vi "Initialize and Enable.vi"(4 "error in (no error)":errorcluster, 7 "axis names":string[](array[string])=["Y", "YY", "X", "Z", "U"]) -> (0 "error out":errorcluster, 3 "controller out":refnum<k24>)   [LabVIEW 2011]
uses:
  C:/Users/Admin/Desktop/Gantry Code Transfer/source/Code Transfer/Aerotech.A3200.dll
  Aerotech.A3200.dll
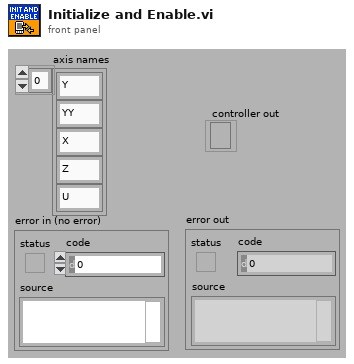
[diagram p1: front panel]
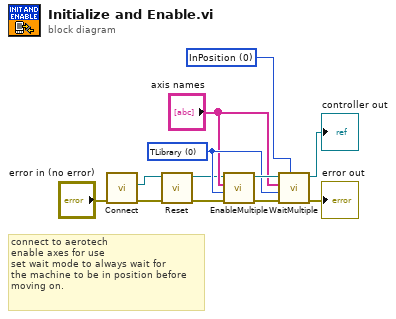
[diagram p0: block diagram]
diagram:
  w11 = 0 items=["InPosition", "MoveDone"] ("wait option?")
  w6 = 0 items=["TLibrary", "T01", "T02", "T03", "T04", "T05", "T06", "T07", "T08", "T09", "T10", "T11", "T12", "T13", "T14", "T15", "T16", "T17", "T18", "T19", "T20", "T21", "T22", "T23", "T24", "T25", "T26", "T27", "T28", "T29", "T30", "T31"] ("taskId")
  # "connect to aerotech\nenable axes for use\nset wait mode to always wait for\nthe machine to be in position before\nmoving on."
  n1 = call "Connect.vi"("error in (no error)"="error in (no error)") -> ("error out"=w3:errorcluster, "controller"=w4:refnum<k24>)  [unwired: 9 in]
  n2 = call "Reset.vi"("error in (no error)"=w3, "controller in"=w4) -> ("error out"=w1:errorcluster, "controller out"=w2:refnum<k24>)  [unwired: 8 in]
  n3 = call "EnableMultiple.vi"("error in (no error)"=w1, "taskId"=w6, "axis names"="axis names", "controller in"=w2) -> ("error out"=w7:errorcluster, "controller out"=w8:refnum<k24>)  [unwired: 6 in]
  n4 = call "WaitMultiple.vi"("wait option?"=w11, "error in (no error)"=w7, "timeout? (msec)"=w6, "axis names"="axis names", "controller in"=w8) -> ("error out"=→"error out":errorcluster, "controller out"=→"controller out":refnum<k24>)  [unwired: 4 in, 1 out]
